vi "Make String Status.vi"(8 "error in (no error)":errorcluster, 11 "Construct String Camera Status in":refnum<class "Construct String Camera Status.lvclass">) -> (0 "error out":errorcluster, 2 "String Camera Status":string, 3 "Construct String Camera Status out":refnum<class "Construct String Camera Status.lvclass">)   [LabVIEW 2018, in "Construct String Camera Status.lvclass"]
doc: "Este VI realiza a leitura das informações salvas na classe, construindo uma string com o status da câmera."
uses:
  Construct String Camera Status.lvclass
  Construct String Camera Status.lvclass/Construct String Camera Status.ctl
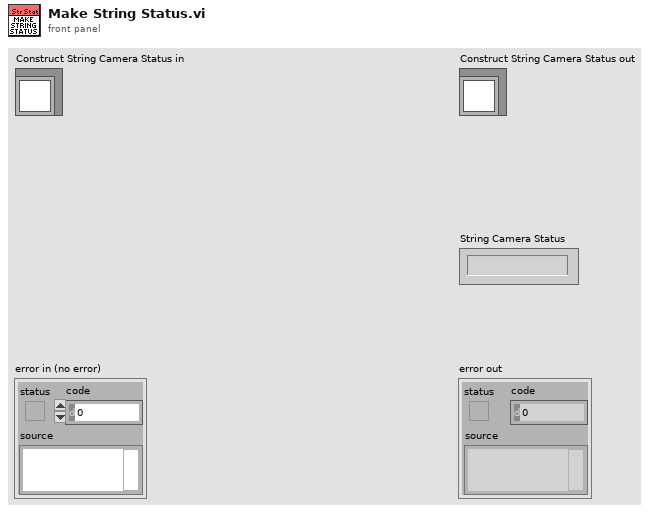
[diagram p1: front panel]
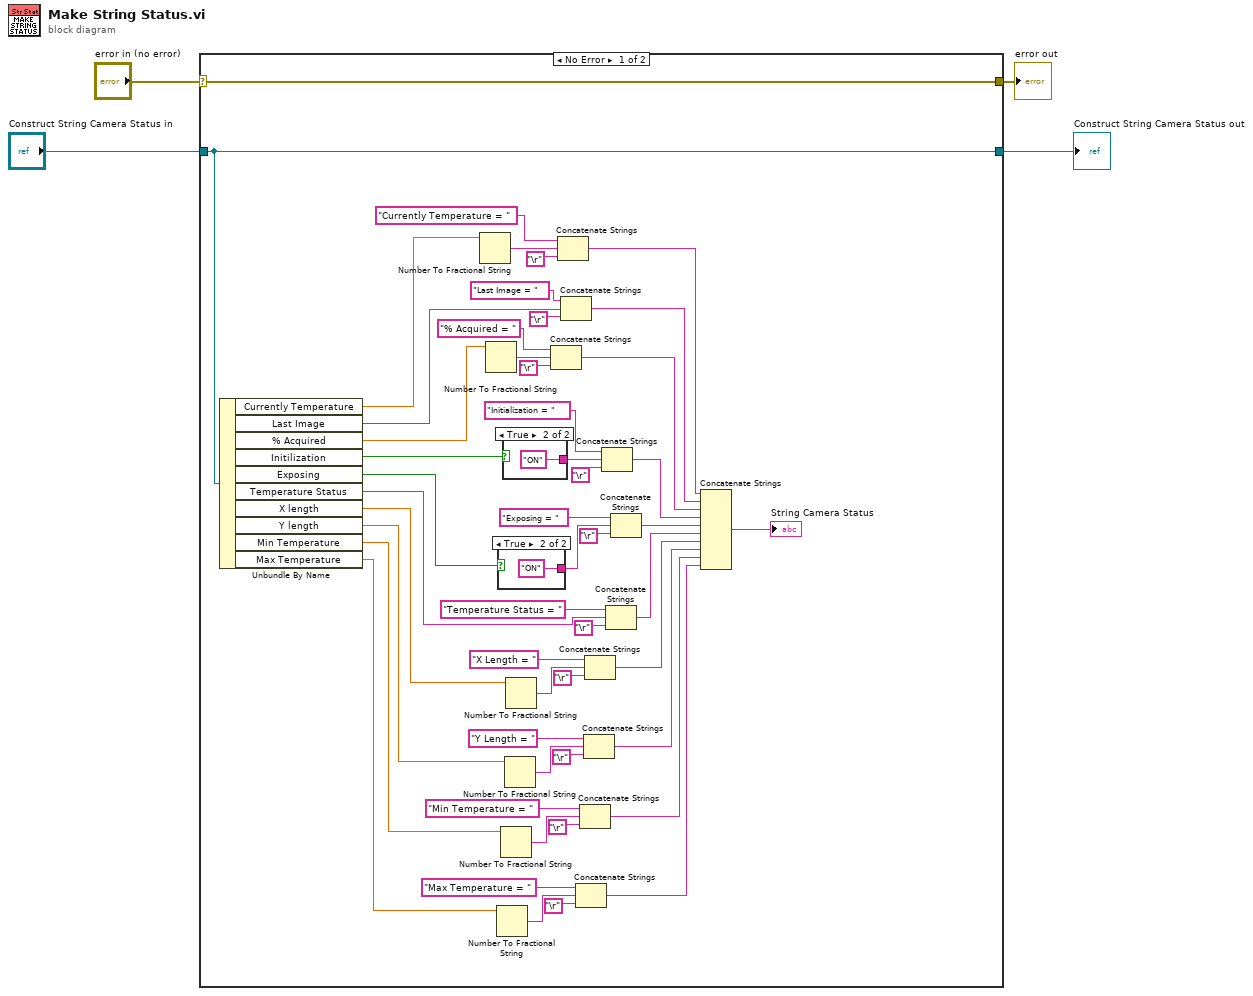
[diagram p0: block diagram]
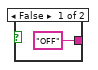
[diagram p2: hidden frame]
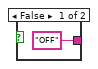
[diagram p3: hidden frame]
diagram:
  n1 = case shown="No Error" "error in (no error)" {
    selector: "error in (no error)" -> [w55 w61]
    tunnel: [w55 w61] -> w3
    tunnel: [w54 w60] -> w1
    tunnel: "Construct String Camera Status in" -> [w54 w60]
    frame No Error {
      n2 = Unbundle By Name(w54) -> ("Currently Temperature"=w53:dbl, "Last Image"=w47:string, "% Acquired"=w44:dbl, "Initilization"=w41:bool, "Exposing"=w40:bool, "Temperature Status"=w33:string, "X length"=w21:dbl, "Y length"=w15:dbl, "Min Temperature"=w11:dbl, "Max Temperature"=w5:dbl)
      n3 = Number To Fractional String(number=w53) -> (F-format string=w51:string)  [unwired: 3 in]
      n4 = Number To Fractional String(number=w44) -> (F-format string=w43:string)  [unwired: 3 in]
      n5 = Number To Fractional String(number=w5) -> (F-format string=w9:string)  [unwired: 3 in]
      n6 = case shown="True" w40 {
        tunnel: ["OFF" "ON"] -> w35
        frame False {
        }
        frame True {
        }
      }
      n7 = Number To Fractional String(number=w11) -> (F-format string=w12:string)  [unwired: 3 in]
      n8 = case shown="True" w41 {
        tunnel: ["OFF" "ON"] -> w39
        frame False {
        }
        frame True {
        }
      }
      n9 = Number To Fractional String(number=w15) -> (F-format string=w19:string)  [unwired: 3 in]
      n10 = Number To Fractional String(number=w21) -> (F-format string=w22:string)  [unwired: 3 in]
      n11 = Concatenate Strings("% Acquired = ", w43, "\r") -> (w29:string)
      n12 = Concatenate Strings("Currently Temperature = ", w51, "\r") -> (w31:string)
      n13 = Concatenate Strings("Last Image = ", w47, "\r") -> (w30:string)
      n14 = Concatenate Strings("Max Temperature = ", w9, "\r") -> (w6:string)
      n15 = Concatenate Strings("Min Temperature = ", w12, "\r") -> (w10:string)
      n16 = Concatenate Strings("Y Length = ", w19, "\r") -> (w16:string)
      n17 = Concatenate Strings("X Length = ", w22, "\r") -> (w20:string)
      n18 = Concatenate Strings("Initialization = ", w39, "\r") -> (w28:string)
      n19 = Concatenate Strings("Temperature Status = ", w33, "\r") -> (w26:string)
      n20 = Concatenate Strings("Exposing = ", w35, "\r") -> (w27:string)
      n21 = Concatenate Strings(w31, w30, w29, w28, w27, w26, w20, w16, w10, w6) -> (→"String Camera Status":string)
    }
    frame Error {
    }
  }
  "error out" <- w3
  "Construct String Camera Status out" <- w1
